vi "老蔡数据库.vi"() -> ()   [LabVIEW 2018]
panel:
  out "error out 4":errorcluster
  out "表格控件":string[][](table)
  out "error out 3":errorcluster
  out "error out 2":errorcluster
  out "error out":errorcluster
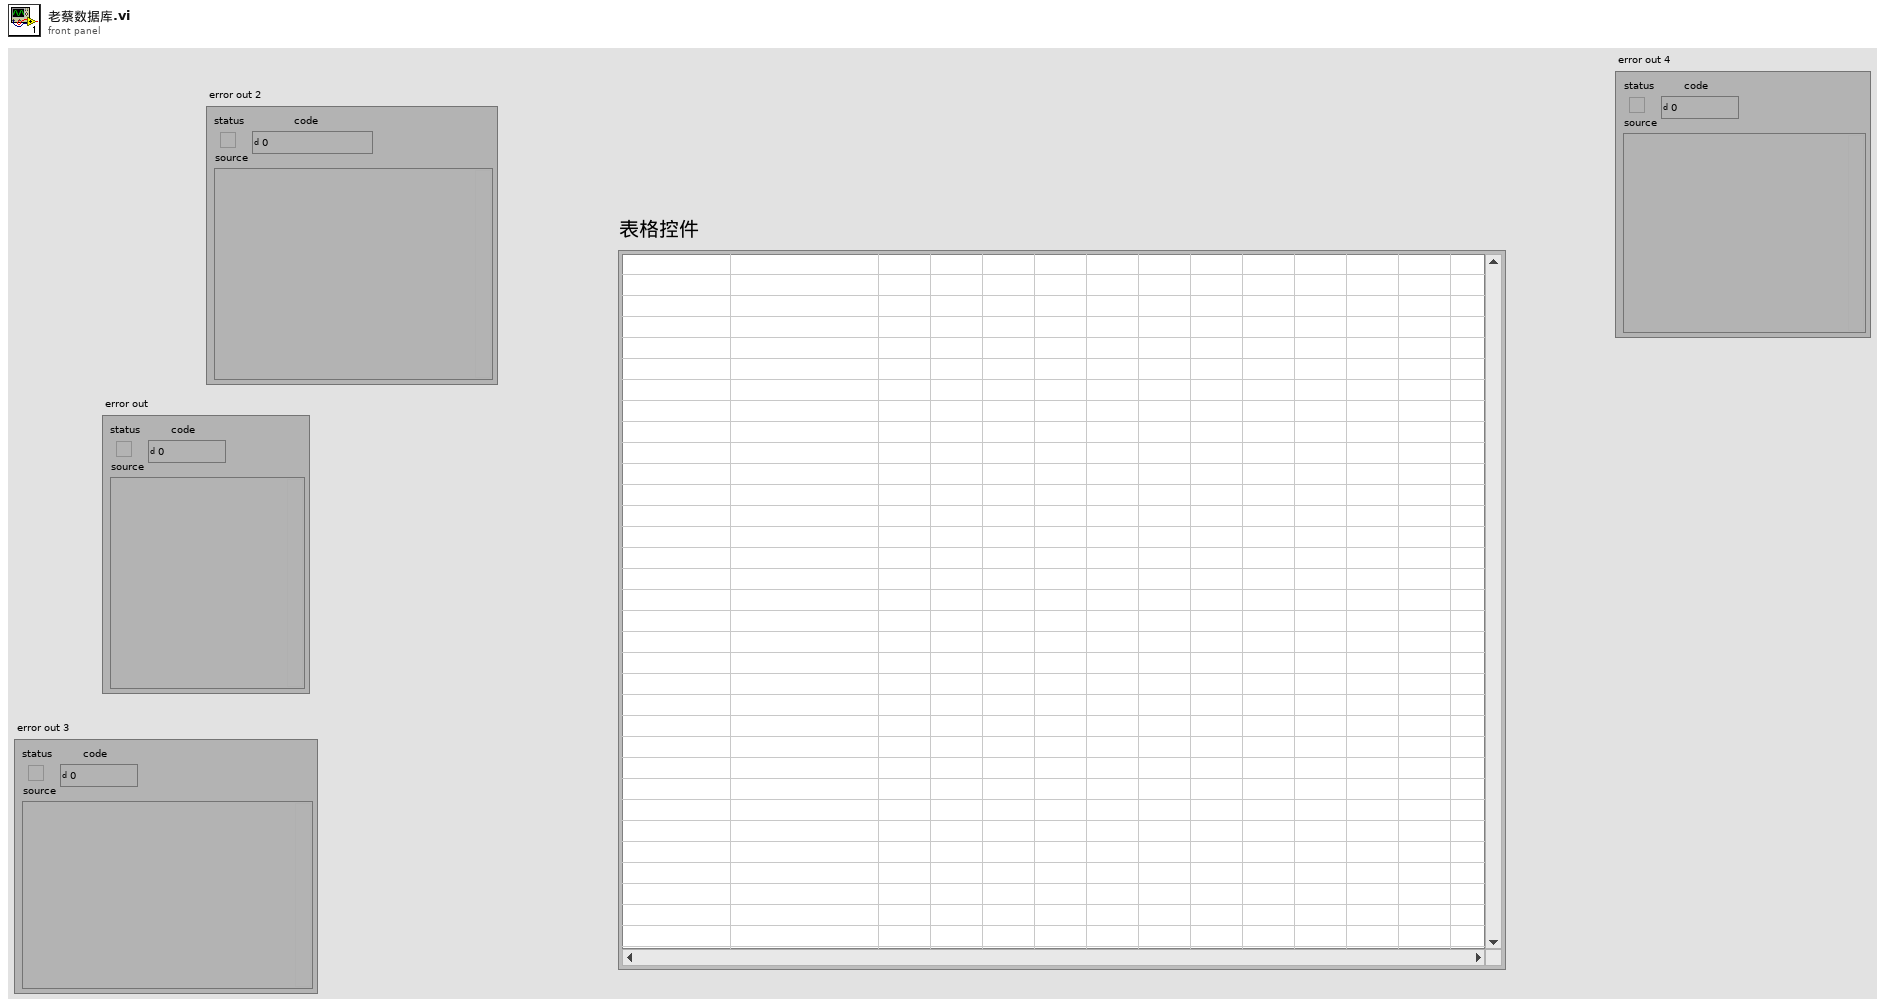
[diagram p1: front panel]
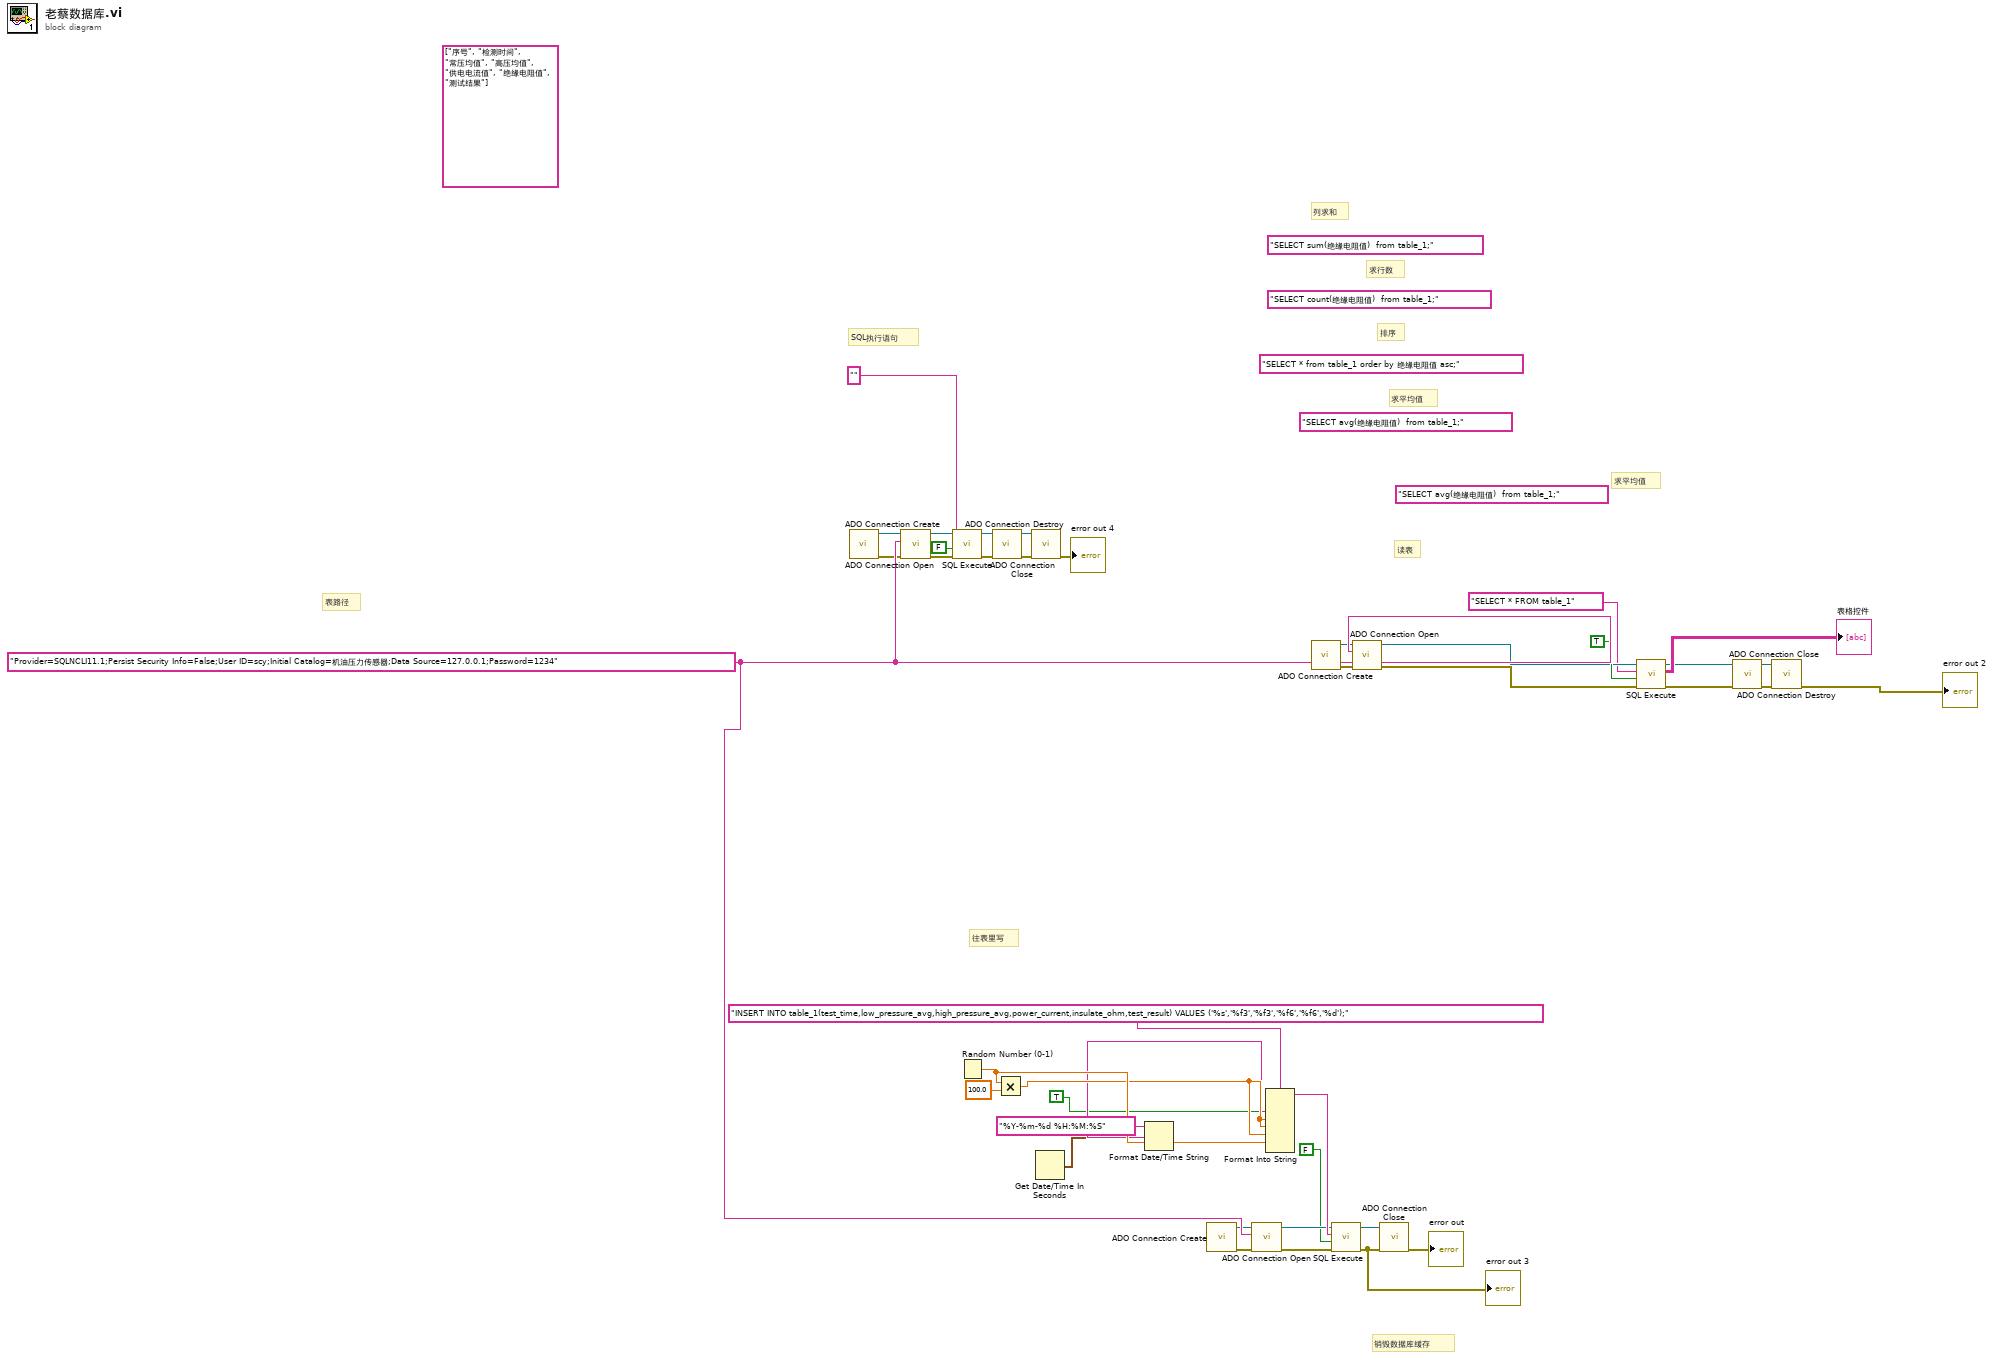
[diagram p0: block diagram]
diagram:
  w41 = "Provider=SQLNCLI11.1;Persist Security Info=False;User ID=scy;Initial Catalog=机油压力传感器;Data Source=127.0.0.1;Password=1234" ("ConnectionString")
  (unwired) "SELECT avg(绝缘电阻值)  from table_1;" ("Command Text")
  (unwired) "SELECT avg(绝缘电阻值)  from table_1;" ("Command Text")
  (unwired) "SELECT * from table_1 order by 绝缘电阻值 asc;" ("Command Text")
  (unwired) "SELECT count(绝缘电阻值)  from table_1;" ("Command Text")
  (unwired) "SELECT sum(绝缘电阻值)  from table_1;" ("Command Text")
  (unwired) string[] ["序号", "检测时间", "常压均值", "高压均值", "供电电流值", "绝缘电阻值", "测试结果"] ("列首字符串[]")
  # "表路径"
  # "往表里写"
  # "读表"
  # "SQL执行语句"
  # "销毁数据库缓存"
  # "求平均值"
  # "排序"
  # "求平均值"
  # "求行数"
  # "列求和"
  n1 = call <userlib>:"ADO Connection Create.vi"() -> ("error out"=w40:errorcluster, "ADODB._Connection Out"=w39:refnum<k7>)  [unwired: 10 in]
  n2 = call <userlib>:"ADO Connection Open.vi"("error in (no error)"=w40, "ConnectionString"=w41, "ADODB._Connection In"=w39) -> ("error out"=w35:errorcluster, "ADODB._Connection Out"=w36:refnum<k7>)  [unwired: 7 in]
  n3 = call <userlib>:"SQL Execute.vi"("error in (no error)"=w35, "Return Data (T)"=FALSE, "Command Text"="", "ADODB._Connection In"=w36) -> ("error out"=w33:errorcluster, "ADODB._Connection Out"=w34:refnum<k7>)  [unwired: 4 in, 2 out]
  n4 = Random Number (0-1)() -> (number: 0 to 1=w29:dbl)
  n5 = call <userlib>:"ADO Connection Close.vi"("error in (no error)"=w33, "ADODB._Connection In"=w34) -> ("error out"=w38:errorcluster, "ADODB._Connection Out"=w37:refnum<k7>)  [unwired: 8 in]
  n6 = Multiply(x=w29, y=100.0) -> (x*y=w28:dbl)
  n7 = call <userlib>:"ADO Connection Destroy.vi"("error in (no error)"=w38, "ADODB._Connection In"=w37) -> ("error out"=→"error out 4":errorcluster)  [unwired: 9 in]
  n8 = Get Date/Time In Seconds() -> (seconds since 1Jan1904=w26:timestamp)
  n9 = Format Date/Time String(time format string (%c)="%Y-%m-%d %H:%M:%S" ("时间格式字符串(%c)"), seconds (now)=w26) -> (date/time string=w27:string)  [unwired: 1 in]
  n10 = call <userlib>:"ADO Connection Create.vi"() -> ("error out"=w18:errorcluster, "ADODB._Connection Out"=w19:refnum<k7>)  [unwired: 10 in]
  n11 = call <userlib>:"ADO Connection Open.vi"("error in (no error)"=w18, "ConnectionString"=w41, "ADODB._Connection In"=w19) -> ("error out"=w24:errorcluster, "ADODB._Connection Out"=w20:refnum<k7>)  [unwired: 7 in]
  n12 = Format Into String(format string="INSERT INTO table_1(test_time,low_pressure_avg,high_pressure_avg,power_current,insulate_ohm,test_result) VALUES ('%s','%f3','%f3','%f6','%f6','%d');", w27, w28, w28, w28, w29, TRUE ("需要秒？(F)")) -> (resulting string=w22:string)  [unwired: 2 in, 1 out]
  n13 = call <userlib>:"ADO Connection Create.vi"() -> ("error out"=w5:errorcluster, "ADODB._Connection Out"=w8:refnum<k7>)  [unwired: 10 in]
  n14 = call <userlib>:"SQL Execute.vi"("error in (no error)"=w24, "Return Data (T)"=FALSE, "Command Text"=w22, "ADODB._Connection In"=w20) -> ("error out"=w25:errorcluster, "ADODB._Connection Out"=w21:refnum<k7>)  [unwired: 4 in, 2 out]
  "error out 3" <- w25
  n15 = call <userlib>:"ADO Connection Open.vi"("error in (no error)"=w5, "ConnectionString"=w41, "ADODB._Connection In"=w8) -> ("error out"=w6:errorcluster, "ADODB._Connection Out"=w9:refnum<k7>)  [unwired: 7 in]
  n16 = call <userlib>:"ADO Connection Close.vi"("error in (no error)"=w25, "ADODB._Connection In"=w21) -> ("error out"=→"error out":errorcluster)  [unwired: 8 in, 1 out]
  n17 = call <userlib>:"SQL Execute.vi"("error in (no error)"=w6, "Return Data (T)"=TRUE, "Command Text"="SELECT * FROM table_1", "ADODB._Connection In"=w9) -> ("error out"=w1:errorcluster, "Data"=→"表格控件":string[][], "ADODB._Connection Out"=w2:refnum<k7>)  [unwired: 4 in, 1 out]
  n18 = call <userlib>:"ADO Connection Close.vi"("error in (no error)"=w1, "ADODB._Connection In"=w2) -> ("error out"=w7:errorcluster, "ADODB._Connection Out"=w10:refnum<k7>)  [unwired: 8 in]
  n19 = call <userlib>:"ADO Connection Destroy.vi"("error in (no error)"=w7, "ADODB._Connection In"=w10) -> ("error out"=→"error out 2":errorcluster)  [unwired: 9 in]
